vi "ReadAll.vi"(4 "Limit":i64, 6 "commandTimeout":i32, 7 "Where":string, 8 "error in (no error)":errorcluster, 9 "DynamicParameters":refnum<class "DynamicParameters.lvclass">, 10 "TableName":string, 11 "SqlMapper in":refnum<class "SqlMapper.lvclass">) -> (0 "error out":errorcluster, 2 "Query Result out":refnum<class "Query Result.lvclass">, 3 "SqlMapper out":refnum<class "SqlMapper.lvclass">)   [LabVIEW 2020, in "ORM.lvlib" / "SqlMapper.lvclass"]
uses:
  SqlMapper.lvclass
  DynamicParameters/DynamicParameters.lvclass
  Query Result/Query Result.lvclass
  SqlMapper.lvclass/SqlMapper.ctl
  DbConnection/DbConnection.lvclass
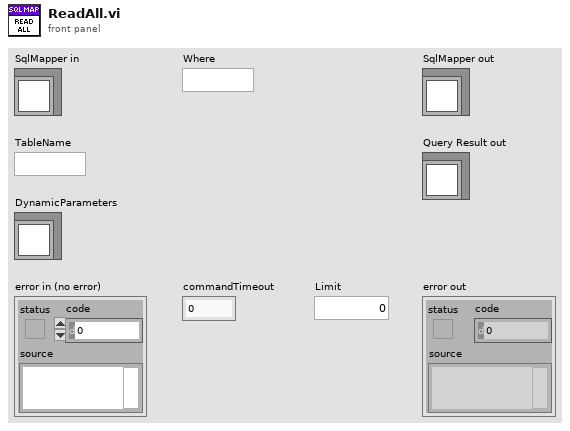
[diagram p1: front panel]
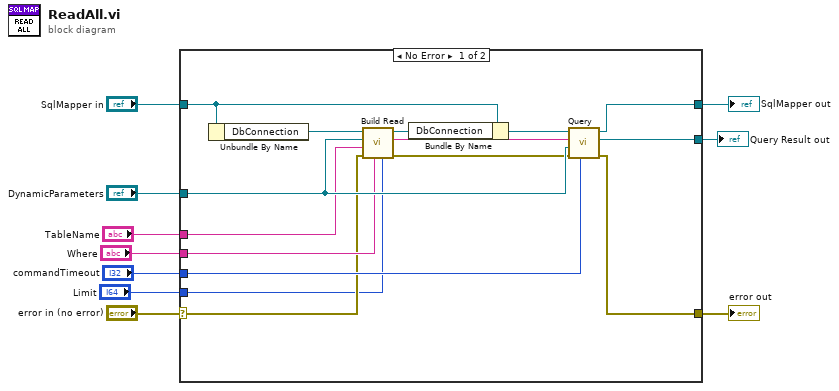
[diagram p0: block diagram]
diagram:
  n1 = case shown="No Error" "error in (no error)" {
    selector: "error in (no error)" -> [w16 w26]
    tunnel: "SqlMapper in" -> [w24 w27]
    tunnel: [w21 w27] -> w8
    tunnel: "commandTimeout" -> [w20 _]
    tunnel: "DynamicParameters" -> [w19 _]
    tunnel: "TableName" -> [w18 _]
    tunnel: "Where" -> [w17 _]
    tunnel: [w14 w26] -> w3
    tunnel: [w13 _] -> w2
    tunnel: "Limit" -> [w11 _]
    frame No Error {
      n2 = Unbundle By Name(w24) -> ("DbConnection"=w25:refnum<class "DbConnection.lvclass">)
      n3 = call-dynamic "Build Read.vi"("Limit"=w11, "Where"=w17, "error in (no error)"=w16, "tableName"=w18, "DynamicParameters in"=w19, "DbConnection in"=w25) -> ("error out"=w15:errorcluster, "Query"=w12:string, "DbConnection out"=w23:refnum<class "DbConnection.lvclass">)  [unwired: 3 in]
      n4 = Bundle By Name(cluster=w24, "DbConnection"=w23) -> (w22:refnum<class "SqlMapper.lvclass">)
      n5 = call-dynamic "Query.vi"("commandTimeout"=w20, "error in (no error)"=w15, "DynamicParameters"=w19, "sql"=w12, "SqlMapper in"=w22) -> ("error out"=w14:errorcluster, "Query Result out"=w13:refnum<class "Query Result.lvclass">, "SqlMapper out"=w21:refnum<class "SqlMapper.lvclass">)  [unwired: 4 in]
    }
    frame Error {
    }
  }
  "error out" <- w3
  "SqlMapper out" <- w8
  "Query Result out" <- w2
